vi "Write Graph Data.vi"(10 "Graph Data":cluster{"Array":dbl[], "Array":dbl[]}[](array[cluster]), 11 "Harmonics in":refnum<class "Harmonics.lvclass">) -> (3 "Harmonics out":refnum<class "Harmonics.lvclass">)   [LabVIEW 2020, in "Harmonics.lvclass"]
uses:
  Harmonics.lvclass
  Harmonics.lvclass/Harmonics.ctl
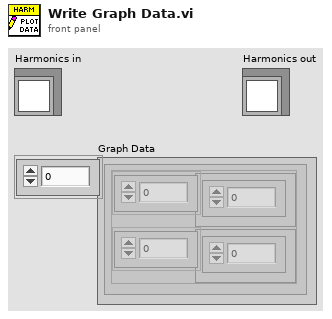
[diagram p1: front panel]
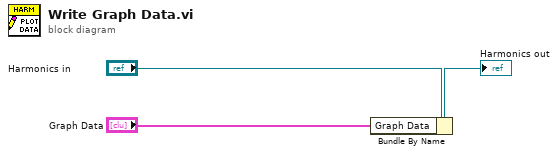
[diagram p0: block diagram]
diagram:
  n1 = Bundle By Name(cluster="Harmonics in", "Graph Data"="Graph Data") -> (→"Harmonics out":refnum<class "Harmonics.lvclass">)
